vi "Write Pretty Print.vi"(8 "error in (no error)":errorcluster, 10 "Pretty Print":bool=TRUE, 11 "Serializer.JDP-JSON in":refnum<class "Serializer.JDP-JSON.lvclass">) -> (0 "error out":errorcluster, 3 "Serializer.JDP-JSON out":refnum<class "Serializer.JDP-JSON.lvclass">)   [LabVIEW 2019, in "OpenSerializer.JDP-JSON.lvlib" / "Serializer.JDP-JSON.lvclass"]
uses:
  Serializer.JDP-JSON.lvclass
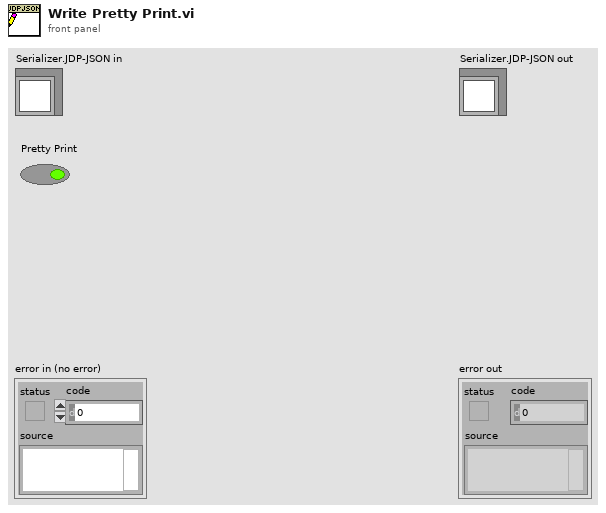
[diagram p1: front panel]
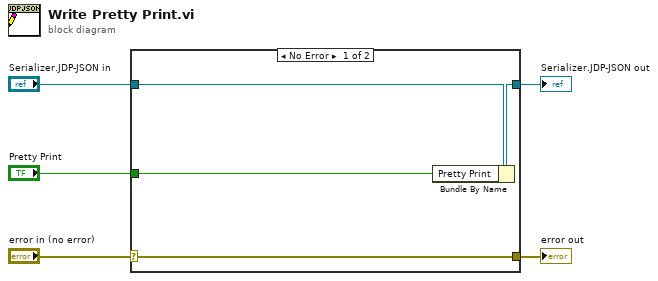
[diagram p0: block diagram]
diagram:
  n1 = case shown="No Error" "error in (no error)" {
    selector: "error in (no error)" -> [w9 w10]
    tunnel: [w9 w10] -> w4
    tunnel: [w7 w11] -> w2
    tunnel: "Serializer.JDP-JSON in" -> [w8 w11]
    tunnel: "Pretty Print" -> [w6 _]
    frame No Error {
      n2 = Bundle By Name(cluster=w8, "Pretty Print"=w6) -> (w7:refnum<class "Serializer.JDP-JSON.lvclass">)
    }
    frame Error {
    }
  }
  "error out" <- w4
  "Serializer.JDP-JSON out" <- w2
